vi "FTW-Test-JSON-Escape.vi"() -> ()   [LabVIEW 2015]
panel:
  out "Elapsed Time 3":dbl format="%.3f sec"
  out "Elapsed Time 2":dbl format="%.3f sec"
  out "Elapsed Time":dbl format="%.3f sec"
  out "Array":string[](array[string])
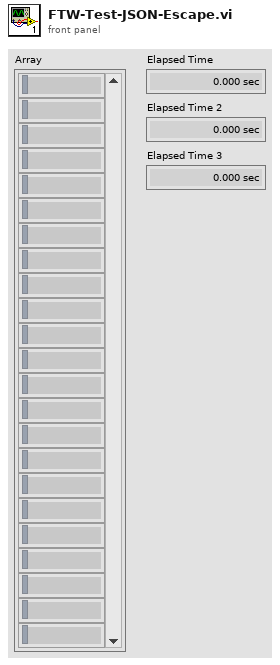
[diagram p1: front panel]
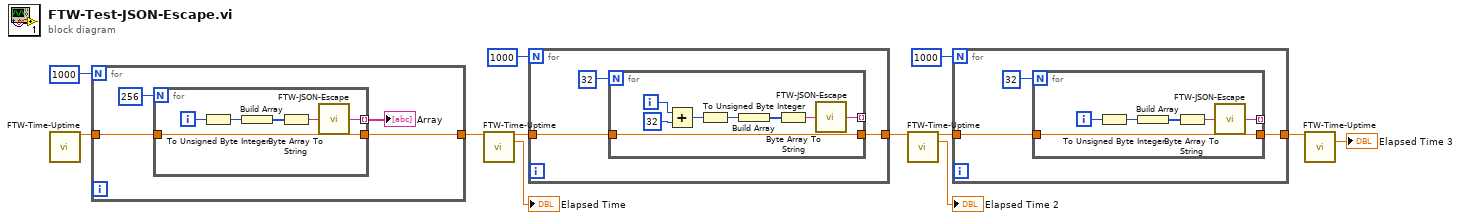
[diagram p0: block diagram]
diagram:
  n1 = call "FTW-Time-Uptime.vi"() -> ("Current Uptime"=w9:dbl)  [unwired: 13 in, 2 out]
  n2 = for {
    N: 1000 -> [_]
    tunnel: [w14] -> w10
    tunnel: w9 -> [w13]
    n3 = for {
      N: 256 -> [_]
      tunnel: [w18] -> w15 mode=indexing
      tunnel: [w17] -> w14
      tunnel: w13 -> [w17]
      i -> [w20]
      n4 = To Unsigned Byte Integer(number=w20) -> (unsigned 8bit integer=w19:u8)
      n5 = Build Array(w19) -> (w22:u8[])
      n6 = Byte Array To String(unsigned byte array=w22) -> (string=w21:string)
      n7 = call "FTW-JSON-Escape.vi"("String"=w21) -> ("Escaped UTF-8 String"=w18:string)
    }
    "Array" <- w15
  }
  n8 = call "FTW-Time-Uptime.vi"("Previous Uptime"=w10) -> ("Current Uptime"=w8:dbl, "Elapsed Time"=→"Elapsed Time":dbl)  [unwired: 12 in, 1 out]
  n9 = for {
    N: 1000 -> [_]
    tunnel: [w24] -> w6
    tunnel: w8 -> [w23]
    n10 = for {
      N: 32 -> [_]
      tunnel: [w29] -> _ mode=indexing
      tunnel: [w28] -> w24
      tunnel: w23 -> [w28]
      i -> [w31]
      n11 = Add(x=w31, y=32 ("x")) -> (x+y=w27:i32)
      n12 = To Unsigned Byte Integer(number=w27) -> (unsigned 8bit integer=w30:u8)
      n13 = Build Array(w30) -> (w33:u8[])
      n14 = Byte Array To String(unsigned byte array=w33) -> (string=w32:string)
      n15 = call "FTW-JSON-Escape.vi"("String"=w32) -> ("Escaped UTF-8 String"=w29:string)
    }
  }
  n16 = call "FTW-Time-Uptime.vi"("Previous Uptime"=w6) -> ("Current Uptime"=w2:dbl, "Elapsed Time"=→"Elapsed Time 2":dbl)  [unwired: 12 in, 1 out]
  n17 = for {
    N: 1000 -> [_]
    tunnel: [w35] -> w3
    tunnel: w2 -> [w34]
    n18 = for {
      N: 32 -> [_]
      tunnel: [w39] -> _ mode=indexing
      tunnel: [w38] -> w35
      tunnel: w34 -> [w38]
      i -> [w37]
      n19 = To Unsigned Byte Integer(number=w37) -> (unsigned 8bit integer=w40:u8)
      n20 = Build Array(w40) -> (w42:u8[])
      n21 = Byte Array To String(unsigned byte array=w42) -> (string=w41:string)
      n22 = call "FTW-JSON-Escape.vi"("String"=w41) -> ("Escaped UTF-8 String"=w39:string)
    }
  }
  n23 = call "FTW-Time-Uptime.vi"("Previous Uptime"=w3) -> ("Elapsed Time"=→"Elapsed Time 3":dbl)  [unwired: 12 in, 2 out]
